vi "PM-Pulse_Measurement-Launcher.vi"() -> ()   [LabVIEW 2018]
uses:
  init-close/PM-init-acquisition_type.ctl
panel:
  in  "Acquisition Instrument":T1
  out "error out":errorcluster
  out "error outprocess":errorcluster
  out "error out aqn":errorcluster
  # "Launcher Press play to start"
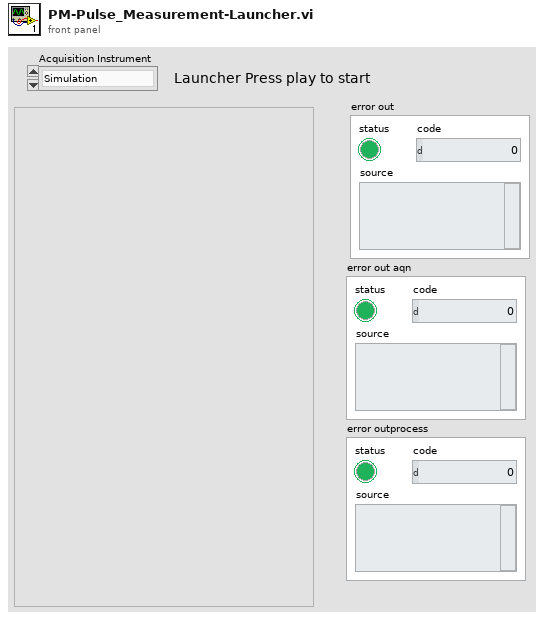
[diagram p1: front panel]
types:
  T1 = typedef "PM-init-acquisition_type.ctl" = enum16{"Simulation", "myDAQ", "Analog Discovery 2", "Arduino/Serial"}
  T2 = typedef "PM-init-data_cluster.ctl" = cluster{"user events":T3}
  T3 = typedef "PM-init-user_events.ctl" = cluster{"stop":refnum<user-event>, "raw wf":refnum<user-event>, "filtered wf":refnum<user-event>, "pulse":refnum<user-event>, "feedback":refnum<user-event>, "raw collected wf":refnum<user-event>, "avg sample size":refnum<user-event>, "Collected sample size":refnum<user-event>, "Post Filtering remove":refnum<user-event>, "Reset avg":refnum<user-event>, "Reset collected wf":refnum<user-event>, "pause aqn":refnum<user-event>, "Peak detect settings":refnum<user-event>}
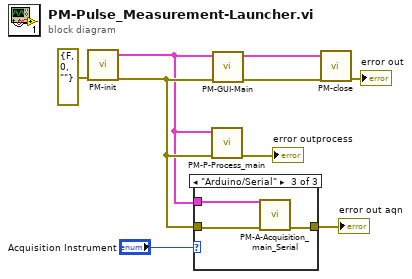
[diagram p0: block diagram]
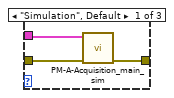
[diagram p2: hidden frame]
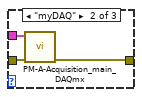
[diagram p3: hidden frame]
diagram:
  n1 = call "PM-init.vi"("error in (no error)"=errorcluster {"status"=FALSE, "code"=0, "source"=""}) -> ("error out"=w9:errorcluster, "init_cluster"=w7:T2)  [unwired: 9 in]
  n2 = case shown="\"Arduino/Serial\"" "Acquisition Instrument" {
    tunnel: w9 -> [w12 w15 w18]
    tunnel: w7 -> [w11 w13 w16]
    tunnel: [w10 w14 w17] -> w5
    frame "Simulation", Default {
      n3 = call "PM-A-Acquisition_main_sim.vi"("error in"=w12, "init_cluster"=w11) -> ("error out"=w10:errorcluster)  [unwired: 9 in]
    }
    frame "myDAQ" {
      n4 = call "PM-A-Acquisition_main_DAQmx.vi"("error in"=w15, "init_cluster"=w13) -> ("error out"=w14:errorcluster)  [unwired: 9 in]
    }
    frame "Arduino/Serial" {
      n5 = call "PM-A-Acquisition_main_Serial.vi"("error in"=w18, "init_cluster"=w16) -> ("error out"=w17:errorcluster)  [unwired: 9 in]
    }
  }
  "error out aqn" <- w5
  n6 = call "PM-P-Process_main.vi"("error out"=w9, "init_cluster"=w7) -> ("error out out"=→"error outprocess":errorcluster)  [unwired: 9 in]
  n7 = call "PM-GUI-Main.vi"("error in"=w9, "init_cluster"=w7) -> ("error out"=w1:errorcluster, "init_cluster out"=w2:T2)  [unwired: 8 in]
  n8 = call "PM-close.vi"("error out"=w1, "init_cluster"=w2) -> ("error out out"=→"error out":errorcluster)  [unwired: 9 in]
